vi "Build Continuous DTC List.vi"(10 "Changed DTCs":T1[](array[typedef]), 11 "Previous Changed DTCs":T1[](array[typedef])) -> (3 "DTCs":T1[](array[typedef]))   [LabVIEW 2013, in "Diagnostics Addon Engine.lvlib"]
uses:
  Diagnostics Addon Engine.lvlib
  Shared/DTC and Timestamp Cluster.ctl
  Shared/Diagnostics Addon Shared.lvlib
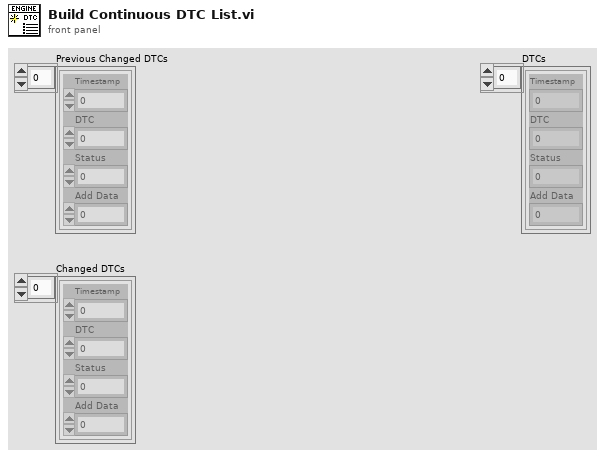
[diagram p1: front panel]
types:
  T1 = typedef "Diagnostics Addon Shared.lvlib/DTC and Timestamp Cluster.ctl" = cluster{"Timestamp":dbl, "DTC":dbl, "Status":dbl, "Add Data":dbl}
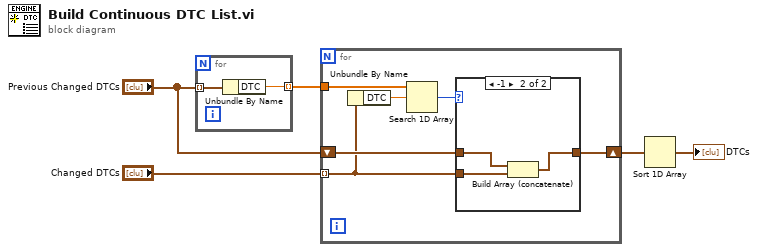
[diagram p0: block diagram]
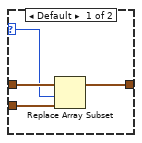
[diagram p2: hidden frame]
diagram:
  n1 = for {
    tunnel: "Previous Changed DTCs" -> [w7] mode=indexing
    tunnel: [w6] -> w5 mode=indexing
    n2 = Unbundle By Name(w7) -> ("DTC"=w6:dbl)
  }
  n3 = for {
    tunnel: "Changed DTCs" -> [w8] mode=indexing
    tunnel: w5 -> [w13]
    shift-right: [w10] -> w4
    shift-left: "Previous Changed DTCs" -> [w11]
    n4 = Unbundle By Name(w8) -> ("DTC"=w9:dbl)
    n5 = Search 1D Array(1D array=w13, element=w9) -> (index of element=w12:i32)  [unwired: 1 in]
    n6 = case shown="-1" w12 {
      selector: w12 -> [w14 _]
      tunnel: w11 -> [w17 w20]
      tunnel: [w16 w19] -> w10
      tunnel: w8 -> [w15 w18]
      frame Default {
        n7 = Replace Array Subset(array=w17, new element=w15, index=w14) -> (w16:T1[])
      }
      frame -1 {
        n8 = Build Array (concatenate)(w20, w18) -> (w19:T1[])
      }
    }
  }
  n9 = Sort 1D Array(array=w4) -> (sorted array=→"DTCs":T1[])
